vi "Execute.OpenSequence.vi"(8 "error in (no error)":errorcluster, 11 "State Variables":T1={"Events.State"=refnum, "Events.Test Result"=refnum, "Events.Progress"=refnum, "INI.Settings"={"Build Location"=path "C:/Simple Sequence Editor/SequenceRepo", "LoggingLocation"=path "", "Sequence.AbortChannel"="", "Sequence.IterationInfoChannel"="", "Sequence.DurationChannel"="", "Sequence.StepInfoChannel"="", "Sequence.SkipChannel"="", "PlotChannels"=[], "Sequence.InitializeScript"=path "C:/Simple Sequence Editor/SequenceRepo", "Sequence.CleanupScript"=path "", "Log.DefaultRate"=0.0}, "NIVS.AlarmManager"=refnum, "NIVS.BaseLogPath"=path "", "NIVS.DataLogManagerRef"=refnum, "NIVS.DataLogSpecRef"=refnum, "NIVS.Deployed"=FALSE, "NIVS.Events"={"SequenceEvent"=refnum, "SystemChangeEvent"=refnum, "WorkspaceEvent"=refnum}, "NIVS.GatewayIPAddress"="", "NIVS.DataLogGUID"="", "NIVS.ProfileCallback"=refnum, "NIVS.ProfileRef"=refnum, "NIVS.SequenceState"=enum."Idle", "NIVS.SystemDefinitionFile"=path "", "NIVS.SystemStateRefs"={"CustDatRef"=refnum, "EvtRef"=refnum, "Target State User Event"=refnum}, "NIVS.WorkspaceManager"=refnum, "NIVS.EventLogGUID"="", "NIVS.EventLogManagerRef"=refnum, "NIVS.EventLogSpecRef"=refnum, "NIVS.BaseToolPath"=path "", "Restart.Path"=path "", "Sequence.#ofColumns"=0, "Sequence.Iterations"=0, "Sequence.Channels"=[], "Sequence.ValidConfig?"=FALSE, "Station.ID"="", "UDP.Queue"=refnum, "UI.Abort"=refnum, "UI.Alarms"=refnum, "UI.Apply"=refnum, "UI.Back"=refnum, "UI.BaseFileName"=refnum, "UI.CurrentIteration"=refnum, "UI.CurrentStep"=refnum, "UI.CyclicFrequency"=refnum, "UI.Description"=refnum, "UI.DelayTime"=refnum, "UI.DisableAlarms"=refnum, "UI.Duration"=refnum, "UI.EnableLogging"=refnum, "UI.EnableState"=refnum, "UI.High"=refnum, "UI.LogChannels"=refnum, "UI.Low"=refnum, "UI.MonitoredVariable"=refnum, "UI.Next"=refnum, "UI.NumberOfCycles"=refnum, "UI.OperatorName"=refnum, "UI.Pause"=refnum, "UI.Profile"=refnum, "UI.Revert"=refnum, "UI.Skip"=refnum, "UI.Start"=refnum, "UI.StartIteration"=refnum, "UI.StartStep"=refnum, "UI.TabControl"=refnum, "UI.TotalIterations"=refnum, "UI.WaveformDefinition"=refnum, "UI.WaveformPreview"=refnum, "UI.WorkOrderNumber"=refnum, "UI.Chart"=refnum, "UI.Status"=refnum, "UI.DataView"=refnum, "UI.Table"=refnum, "UI.Multihead"=refnum, "UI.ToolTab"=refnum, "UI.Result"=refnum, "UI.Log Path"=refnum, "UI.ReportPath"=refnum, "UI.RestartPath"=refnum, "UI.AlarmLog"=refnum}) -> (0 "error out":errorcluster)   [LabVIEW 2015, in "Single Station Execution.lvlib"]
uses:
  Single Station Execution.lvlib
  Types/Main.StateVariables.ctl
  Types/INI.Settings.ctl
  <vilib>/NI Veristand/Execution/AlarmManager/AlarmManagerAPI.ctl
  NationalInstruments.VeriStand.ClientAPI
  <vilib>/NI Veristand/Execution/DataLogging/IDataLogging Ref.ctl
  <vilib>/NI Veristand/Execution/DataLogging/DataLoggingSpecification Ref.ctl
  Types/Execute.UserEventRefs.ctl
  <vilib>/NI Veristand/Execution/Workspace/SystemStateRegEventRef.ctl
  <vilib>/NI Veristand/Execution/Workspace/Target State Info.ctl
  <vilib>/NI Veristand/Execution/Workspace/Target State.ctl
  NationalInstruments.VeriStand.RealTimeSequenceDefinitionApi
  Types/Execution.SequenceState.ctl
  <vilib>/NI Veristand/Execution/Workspace/SystemStateEventRef.ctl
  <vilib>/NI Veristand/Execution/Workspace/WorkspaceAPI.ctl
  Types/UDPEngine.QueueCluster.ctl
  Types/UDPEngine.State.ctl
  <vilib>/NI Veristand/Execution/Workspace/NI_VS Workspace ExecutionAPI.lvlib
  <vilib>/NI Veristand/Execution/DataLogging/NI_VS Data Logging API.lvlib
  <vilib>/NI Veristand/Execution/AlarmManager/NI_VS AlarmManager ExecutionAPI.lvlib
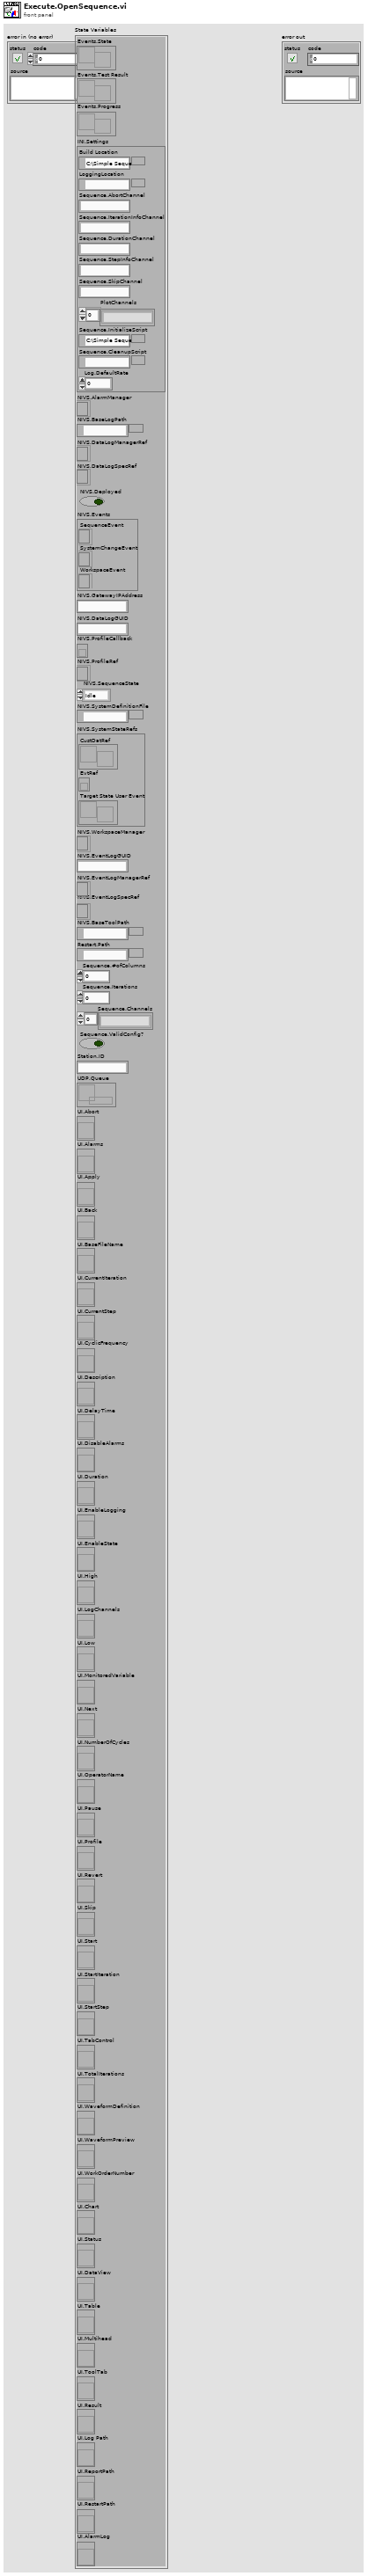
[diagram p1: front panel]
types:
  T1 = typedef "Single Station Execution.lvlib/Main.StateVariables.ctl" = cluster{"Events.State":refnum<user-event>, "Events.Test Result":refnum<user-event>, "Events.Progress":refnum<user-event>, "INI.Settings":T2, "NIVS.AlarmManager":T3, "NIVS.BaseLogPath":path, "NIVS.DataLogManagerRef":T4, "NIVS.DataLogSpecRef":T5, "NIVS.Deployed":bool, "NIVS.Events":T6, "NIVS.GatewayIPAddress":string, "NIVS.DataLogGUID":string, "NIVS.ProfileCallback":refnum<k27>, "NIVS.ProfileRef":refnum<k24>, "NIVS.SequenceState":T8, "NIVS.SystemDefinitionFile":path, "NIVS.SystemStateRefs":T9, "NIVS.WorkspaceManager":T10, "NIVS.EventLogGUID":string, "NIVS.EventLogManagerRef":T4, "NIVS.EventLogSpecRef":T5, "NIVS.BaseToolPath":path, "Restart.Path":path, "Sequence.#ofColumns":i32, "Sequence.Iterations":u32, "Sequence.Channels":string[], "Sequence.ValidConfig?":bool, "Station.ID":string, "UDP.Queue":refnum<queue>, "UI.Abort":refnum<vi>, "UI.Alarms":refnum<vi>, "UI.Apply":refnum<vi>, "UI.Back":refnum<vi>, "UI.BaseFileName":refnum<vi>, "UI.CurrentIteration":refnum<vi>, "UI.CurrentStep":refnum<vi>, "UI.CyclicFrequency":refnum<vi>, "UI.Description":refnum<vi>, "UI.DelayTime":refnum<vi>, "UI.DisableAlarms":refnum<vi>, "UI.Duration":refnum<vi>, "UI.EnableLogging":refnum<vi>, "UI.EnableState":refnum<vi>, "UI.High":refnum<vi>, "UI.LogChannels":refnum<vi>, "UI.Low":refnum<vi>, "UI.MonitoredVariable":refnum<vi>, "UI.Next":refnum<vi>, "UI.NumberOfCycles":refnum<vi>, "UI.OperatorName":refnum<vi>, "UI.Pause":refnum<vi>, "UI.Profile":refnum<vi>, "UI.Revert":refnum<vi>, "UI.Skip":refnum<vi>, "UI.Start":refnum<vi>, "UI.StartIteration":refnum<vi>, "UI.StartStep":refnum<vi>, "UI.TabControl":refnum<vi>, "UI.TotalIterations":refnum<vi>, "UI.WaveformDefinition":refnum<vi>, "UI.WaveformPreview":refnum<vi>, "UI.WorkOrderNumber":refnum<vi>, "UI.Chart":refnum<vi>, "UI.Status":refnum<vi>, "UI.DataView":refnum<vi>, "UI.Table":refnum<vi>, "UI.Multihead":refnum<vi>, "UI.ToolTab":refnum<vi>, "UI.Result":refnum<vi>, "UI.Log Path":refnum<vi>, "UI.ReportPath":refnum<vi>, "UI.RestartPath":refnum<vi>, "UI.AlarmLog":refnum<vi>}
  T2 = typedef "Single Station Execution.lvlib/INI.Settings.ctl" = cluster{"Build Location":path, "LoggingLocation":path, "Sequence.AbortChannel":string, "Sequence.IterationInfoChannel":string, "Sequence.DurationChannel":string, "Sequence.StepInfoChannel":string, "Sequence.SkipChannel":string, "PlotChannels":string[], "Sequence.InitializeScript":path, "Sequence.CleanupScript":path, "Log.DefaultRate":dbl}
  T3 = typedef "NI_VS AlarmManager ExecutionAPI.lvlib/AlarmManagerAPI.ctl" = refnum<k24>
  T4 = typedef "NI_VS Data Logging API.lvlib/IDataLogging Ref.ctl" = refnum<k24>
  T5 = typedef "NI_VS Data Logging API.lvlib/DataLoggingSpecification Ref.ctl" = refnum<k24>
  T6 = typedef "Single Station Execution.lvlib/Execute.UserEventRefs.ctl" = cluster{"SequenceEvent":refnum<event-registration>, "SystemChangeEvent":T7, "WorkspaceEvent":refnum<event-registration>}
  T7 = typedef "NI_VS Workspace ExecutionAPI.lvlib/SystemStateRegEventRef.ctl" = refnum<event-registration>
  T8 = typedef "Single Station Execution.lvlib/Execution.SequenceState.ctl" = enum16{"Idle", "Initializing", "Running", "Paused", "Finalizing", "Complete"}
  T9 = typedef "NI_VS Workspace ExecutionAPI.lvlib/SystemStateEventRef.ctl" = cluster{"CustDatRef":refnum<user-event>, "EvtRef":refnum<k27>, "Target State User Event":refnum<user-event>}
  T10 = typedef "NI_VS Workspace ExecutionAPI.lvlib/WorkspaceAPI.ctl" = refnum<k24>
  T11 = enum8{"Enabled", "Disabled", "Disabled and Grayed Out"}
  T12 = typedef "Single Station Execution.lvlib/Restart.Settings.ctl" = cluster{"LogFile":path, "Log Settings":T13[], "StimulusProfile":path, "StopIteration":u32, "StopStep":u32, "Log Channels":T17, "Base File Name":string, "Enable Logging":bool, "Profile":string, "StopDuration":dbl, "Waveform Definition":path, "Number of Cycles":dbl, "Cyclic Frequency":dbl, "Work Order Number":string, "Operator Name":string, "Description":string, "Station.ID":string, "Sequence.Channels":string[], "Alarms":T18[]}
  T13 = typedef "NI_VS Data Logging API.lvlib/TDMS Channel Group.ctl" = cluster{"Group Name":string, "Group Description":string, "Group Properties":T14[], "Channels":T15[], "Time Channel Options":T16, "Time Channel Name":string}
  T14 = typedef "NI_VS Data Logging API.lvlib/TDMS Property.ctl" = cluster{"Name":string, "Value":variant}
  T15 = typedef "NI_VS Data Logging API.lvlib/TDMS Channel.ctl" = cluster{"Channel Name":string, "Channel Path":string, "Channel Description":string, "Channel Properties":T14[]}
  T16 = typedef "NI_VS Data Logging API.lvlib/Time Channel Options.ctl" = enum16{"No Time Channel", "Absolute Time", "System Time", "System Time - Microseconds", "Absolute Time as Double", "Relative To First Start Trigger", "Relative To Session Start"}
  T17 = typedef "Single Station Execution.lvlib/Log.SelectedChannels.ctl" = enum16{"Channels (No System Channel)", "Aliases", "All"}
  T18 = typedef "Single Station Execution.lvlib/Config.AlarmSettings.ctl" = cluster{"Watch Channel":string, "High Limit":dbl, "Low Limit":dbl, "Delay":dbl, "State":enum16{"Disabled", "Enabled", "Tripped", "Delayed Trip", "Indicate"}, "Alarm Name":string}
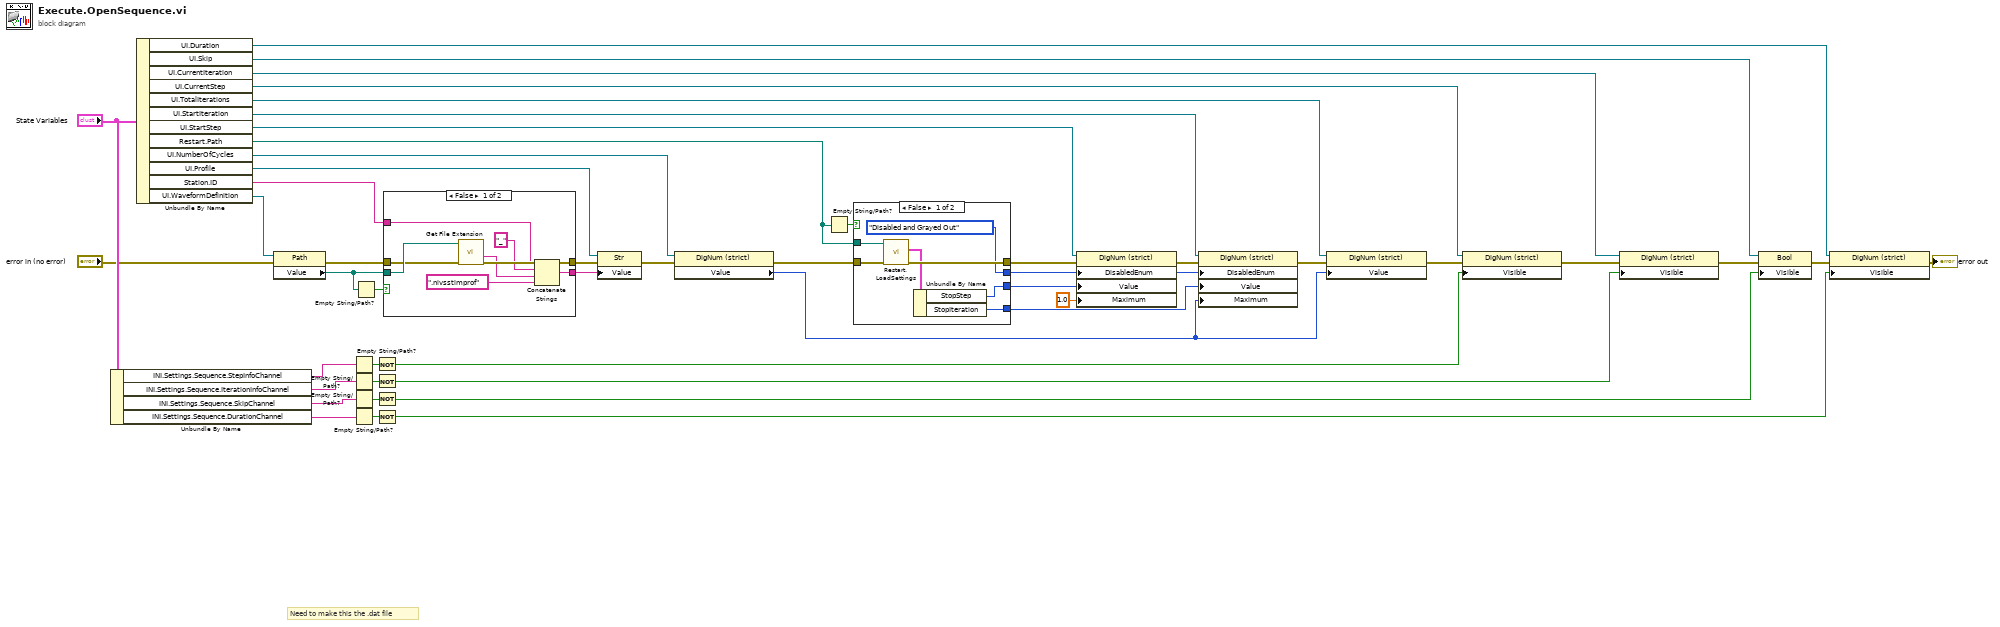
[diagram p0: block diagram]
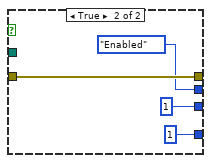
[diagram p3: hidden frame]
diagram:
  # "Need to make this the .dat file"
  n1 = Unbundle By Name("State Variables") -> ("INI.Settings.Sequence.StepInfoChannel"=w18:string, "INI.Settings.Sequence.IterationInfoChannel"=w17:string, "INI.Settings.Sequence.SkipChannel"=w16:string, "INI.Settings.Sequence.DurationChannel"=w15:string)
  n2 = Unbundle By Name("State Variables") -> ("UI.Duration"=w21:refnum<vi>, "UI.Skip"=w33:refnum<vi>, "UI.CurrentIteration"=w44:refnum<vi>, "UI.CurrentStep"=w45:refnum<vi>, "UI.TotalIterations"=w37:refnum<vi>, "UI.StartIteration"=w47:refnum<vi>, "UI.StartStep"=w41:refnum<vi>, "Restart.Path"=w29:path, "UI.NumberOfCycles"=w14:refnum<vi>, "UI.Profile"=w7:refnum<vi>, "Station.ID"=w1:string, "UI.WaveformDefinition"=w10:refnum<vi>)
  n3 = property class="Path"(reference=w10, error in="error in (no error)") -> (error out=w8:errorcluster, "Value"=w2:path)  [unwired: 1 out]
  n4 = Empty String/Path?(string/path=w18) -> (empty?=w42:bool)
  n5 = Empty String/Path?(string/path=w17) -> (empty?=w43:bool)
  n6 = Empty String/Path?(string/path=w16) -> (empty?=w32:bool)
  n7 = Empty String/Path?(string/path=w15) -> (empty?=w25:bool)
  n8 = Empty String/Path?(string/path=w2) -> (empty?=w3:bool)
  n9 = Not(x=w42) -> (.not. x?=w36:bool)
  n10 = Not(x=w43) -> (.not. x?=w35:bool)
  n11 = Not(x=w32) -> (.not. x?=w31:bool)
  n12 = Not(x=w25) -> (.not. x?=w22:bool)
  n13 = case shown="False" w3 {
    tunnel: w2 -> [w55 _]
    tunnel: w8 -> [w54 w56]
    tunnel: [w53 w56] -> w6
    tunnel: [w50 _] -> w4
    tunnel: w1 -> [w48 _]
    frame False {
      n14 = call <vilib>:"Get File Extension.vi"("error in (no error)"=w54, "file"=w55) -> ("error out"=w53:errorcluster, "filename without extension"=w52:string)  [unwired: 5 in, 3 out]
      n15 = Concatenate Strings(w48, "_" ("string"), w52, ".nivsstimprof" ("string")) -> (w50:string)
    }
    frame True {
    }
  }
  n16 = property class="Str"(reference=w7, error in=w6, "Value"=w4) -> (error out=w5:errorcluster)  [unwired: 1 out]
  n17 = property class="DigNum (strict)"(reference=w14, error in=w5) -> (error out=w11:errorcluster, "Value"=w13:u32)  [unwired: 1 out]
  n18 = Empty String/Path?(string/path=w29) -> (empty?=w28:bool)
  n19 = case shown="False" w28 {
    tunnel: w11 -> [w63 w65]
    tunnel: [w62 w65] -> w30
    tunnel: w29 -> [w61 _]
    tunnel: [w58 u32 1 ("Value")] -> w27
    tunnel: [w59 u32 1 ("Value")] -> w26
    tunnel: [T11."Disabled and Grayed Out" ("Disabled") T11."Enabled" ("Disabled")] -> w20
    frame False {
      n20 = call "Restart.LoadSettings.vi"("error in"=w63, "path (use dialog)"=w61) -> ("error out"=w62:errorcluster, "Restart Settings"=w60:T12)  [unwired: 7 in, 1 out]
      n21 = Unbundle By Name(w60) -> ("StopStep"=w58:u32, "StopIteration"=w59:u32)
    }
    frame True {
    }
  }
  n22 = property class="DigNum (strict)"(reference=w41, error in=w30, "DisabledEnum"=w20, "Value"=w27, "Maximum"=1.0 ("Data Entry Limits:Maximum")) -> (error out=w40:errorcluster)  [unwired: 1 out]
  n23 = property class="DigNum (strict)"(reference=w47, error in=w40, "DisabledEnum"=w20, "Value"=w26, "Maximum"=w13) -> (error out=w39:errorcluster)  [unwired: 1 out]
  n24 = property class="DigNum (strict)"(reference=w37, error in=w39, "Value"=w13) -> (error out=w38:errorcluster)  [unwired: 1 out]
  n25 = property class="DigNum (strict)"(reference=w45, error in=w38, "Visible"=w36) -> (error out=w46:errorcluster)  [unwired: 1 out]
  n26 = property class="DigNum (strict)"(reference=w44, error in=w46, "Visible"=w35) -> (error out=w34:errorcluster)  [unwired: 1 out]
  n27 = property class="Bool"(reference=w33, error in=w34, "Visible"=w31) -> (error out=w24:errorcluster)  [unwired: 1 out]
  n28 = property class="DigNum (strict)"(reference=w21, error in=w24, "Visible"=w22) -> (error out=→"error out":errorcluster)  [unwired: 1 out]
